vi "SetConfig.vi"(6 "ID":string, 8 "error in (no error)":errorcluster, 9 "Port":u16, 10 "Address":string, 11 "ClientBase in":refnum<class "ClientBase.lvclass">) -> (0 "error out":errorcluster, 3 "ClientBase out":refnum<class "ClientBase.lvclass">)   [LabVIEW 2020, in "ClientBaseLib.lvlib" / "ClientBase.lvclass"]
uses:
  ClientBase.lvclass
  ClientBase.lvclass/ClientBase.ctl
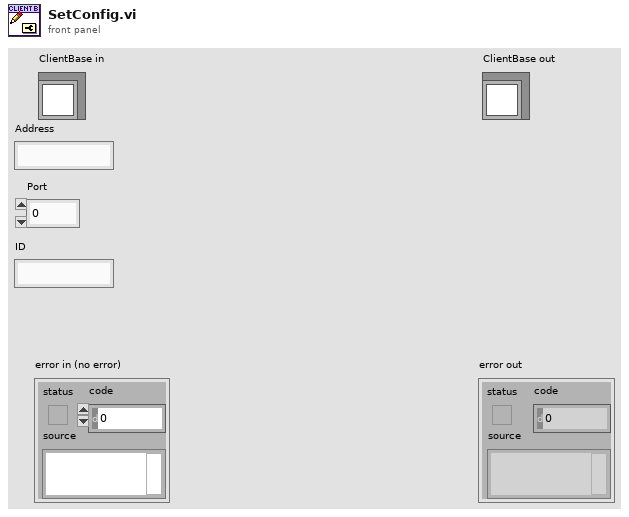
[diagram p1: front panel]
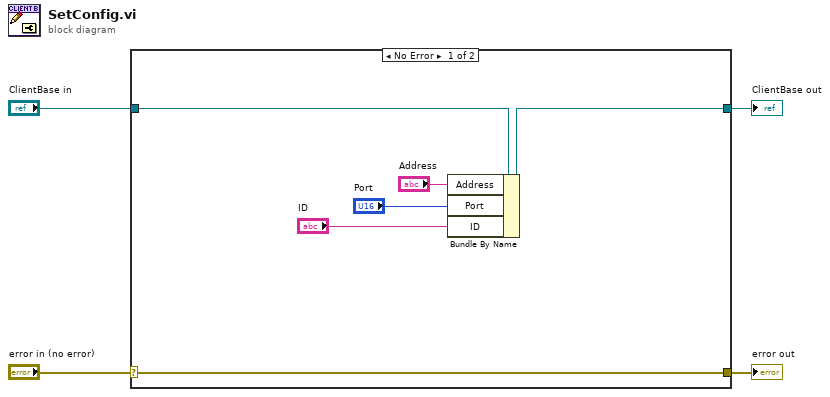
[diagram p0: block diagram]
diagram:
  n1 = case shown="No Error" "error in (no error)" {
    selector: "error in (no error)" -> [w9 w12]
    tunnel: [w9 w12] -> w3
    tunnel: [w8 w11] -> w1
    tunnel: "ClientBase in" -> [w10 w11]
    frame No Error {
      n2 = Bundle By Name(cluster=w10, "Address"="Address", "Port"="Port", "ID"="ID") -> (w8:refnum<class "ClientBase.lvclass">)
    }
    frame Error {
    }
  }
  "error out" <- w3
  "ClientBase out" <- w1
